vi "Check Conditions.vi"(7 "Reset":bool, 8 "Height":dbl, 9 "Dist":dbl, 11 "Condition":i32) -> (3 "Done?":bool)   [LabVIEW 2014]
uses:
  Robot Global Data.vi
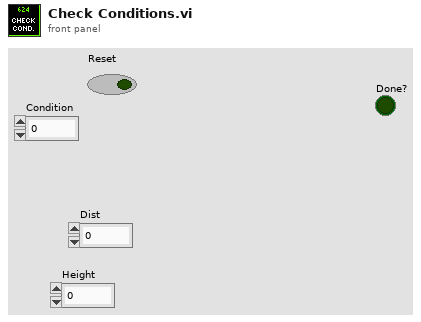
[diagram p1: front panel]
types:
  T1 = typedef "Elevator Status.ctl" = cluster{"Height":dbl, "Enc Value":dbl, "Limit Override":bool, "Mode":T2, "High IR":bool, "Motor Out":dbl, "Ping Detect":bool, "Auto Elevator Indicators":T3, "Master Current":dbl, "Slave Current":dbl, "High Current":bool, "Current Tripped":bool, "Top Limit":bool, "Bottom Limit":bool, "Eject Piston":bool, "Stabilizer":bool, "Finger":bool, "Finger Height":dbl, "Finger Raw":dbl, "Finger at Bottom":bool}
  T2 = typedef "Elevator Mode.ctl" = enum16{"Manual", "Safe", "Auto"}
  T3 = typedef "Auto Elevator Indicators.ctl" = cluster{"Target Out":dbl, "Storing Trashcan?":bool, "State":T4, "In Range":bool, "Store Can Command":bool, "HP Load":bool}
  T4 = typedef "Elevator State.ctl" = enum16{"Idle", "Goto Load Position", "Wait for Load", "Load Drop", "Load Lift", "Drop Stack", "Goto Eject Position", "Eject ", "Raise Trashcan", "Open Stabilizer", "Untip Drop", "Untip Wait", "Untip Lift", "Abort Load", "HP Load Wait", "HP Load Drop", "HP Load Lift", "HP Load Abort", "Close Stabilizer", "HP Load Unfinish", "HP Load Score", "HP Load Finish", "HP Goto Finish Down", "HP Goto Finish Up", "Full"}
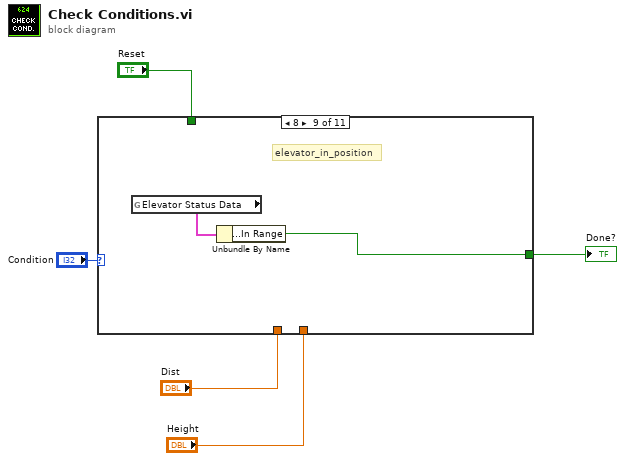
[diagram p0: block diagram]
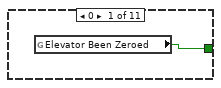
[diagram p2: hidden frame]
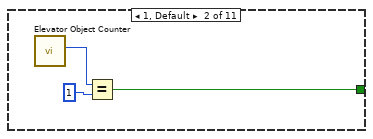
[diagram p3: hidden frame]
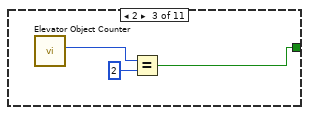
[diagram p4: hidden frame]
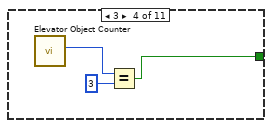
[diagram p5: hidden frame]
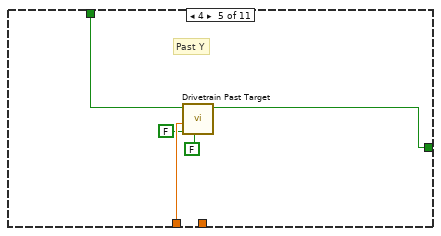
[diagram p6: hidden frame]
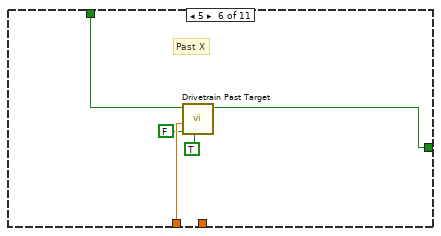
[diagram p7: hidden frame]
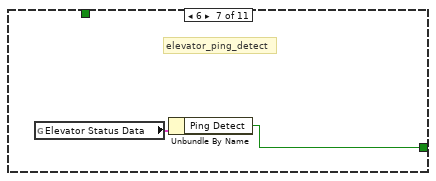
[diagram p8: hidden frame]
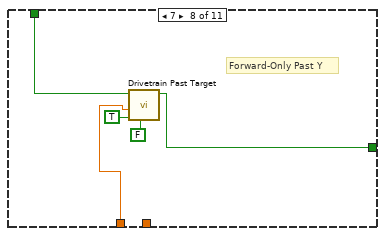
[diagram p9: hidden frame]
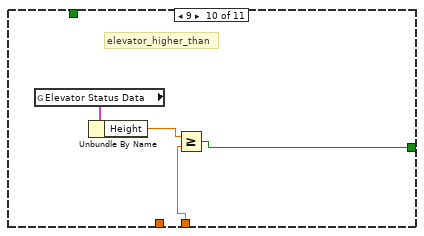
[diagram p10: hidden frame]
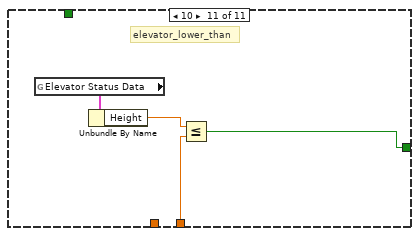
[diagram p11: hidden frame]
diagram:
  n1 = case shown="8" "Condition" {
    tunnel: [w6 w7 w10 w13 w20 w25 w26 w28 w33 w35 w39] -> w4
    tunnel: "Reset" -> [_ _ _ _ w19 w24 _ w30 _ _ _]
    tunnel: "Dist" -> [_ _ _ _ w17 w22 _ w29 _ _ _]
    tunnel: "Height" -> [_ _ _ _ _ _ _ _ _ w36 w40]
    frame 0 {
      n2 = global read "Robot Global Data.vi" "Elevator Been Zeroed"() -> (w6:bool)
    }
    frame 1, Default {
      n3 = call "Elevator Object Counter.vi"() -> ("Tote Count"=w9:i8)  [unwired: 10 in, 1 out]
      n4 = Equal?(x=w9, y=i8 1) -> (x = y?=w7:bool)
    }
    frame 2 {
      n5 = call "Elevator Object Counter.vi"() -> ("Tote Count"=w11:i8)  [unwired: 10 in, 1 out]
      n6 = Equal?(x=w11, y=i8 2) -> (x = y?=w10:bool)
    }
    frame 3 {
      n7 = call "Elevator Object Counter.vi"() -> ("Tote Count"=w14:i8)  [unwired: 10 in, 1 out]
      n8 = Equal?(x=w14, y=i8 3) -> (x = y?=w13:bool)
    }
    frame 4 {
      # "Past Y"
      n9 = call "Drivetrain Past Target.vi"("Use X Distance?"=FALSE, "Forward Only?"=FALSE, "Distance Target"=w17, "Reset"=w19) -> ("Past Target?"=w20:bool)  [unwired: 7 in]
    }
    frame 5 {
      # "Past X"
      n10 = call "Drivetrain Past Target.vi"("Use X Distance?"=TRUE, "Forward Only?"=FALSE, "Distance Target"=w22, "Reset"=w24) -> ("Past Target?"=w25:bool)  [unwired: 7 in]
    }
    frame 6 {
      # "elevator_ping_detect"
      n11 = global read "Robot Global Data.vi" "Elevator Status Data"() -> (w27:T1)
      n12 = Unbundle By Name(w27) -> ("Ping Detect"=w26:bool)
    }
    frame 7 {
      # "Forward-Only Past Y"
      n13 = call "Drivetrain Past Target.vi"("Use X Distance?"=FALSE, "Forward Only?"=TRUE, "Distance Target"=w29, "Reset"=w30) -> ("Past Target?"=w28:bool)  [unwired: 7 in]
    }
    frame 8 {
      # "elevator_in_position"
      n14 = global read "Robot Global Data.vi" "Elevator Status Data"() -> (w34:T1)
      n15 = Unbundle By Name(w34) -> ("Auto Elevator Indicators.In Range"=w33:bool)
    }
    frame 9 {
      # "elevator_higher_than"
      n16 = global read "Robot Global Data.vi" "Elevator Status Data"() -> (w38:T1)
      n17 = Unbundle By Name(w38) -> ("Height"=w37:dbl)
      n18 = Greater Or Equal?(x=w37, y=w36) -> (x >= y?=w35:bool)
    }
    frame 10 {
      # "elevator_lower_than"
      n19 = global read "Robot Global Data.vi" "Elevator Status Data"() -> (w42:T1)
      n20 = Unbundle By Name(w42) -> ("Height"=w41:dbl)
      n21 = Less Or Equal?(x=w41, y=w40) -> (x <= y?=w39:bool)
    }
  }
  "Done?" <- w4
